vi "is_valid_ref.vi"(7 "raise error if invalid? (False)":bool, 8 "error in (no error)":errorcluster, 11 "Table in":refnum<class "Table.lvclass">) -> (0 "error out":errorcluster, 2 "is_valid_ref?":bool, 3 "Table out":refnum<class "Table.lvclass">)   [LabVIEW 2020, in "toml_edit.lvlib" / "Table.lvclass"]
uses:
  Table.lvclass
  Table.lvclass/Table.ctl
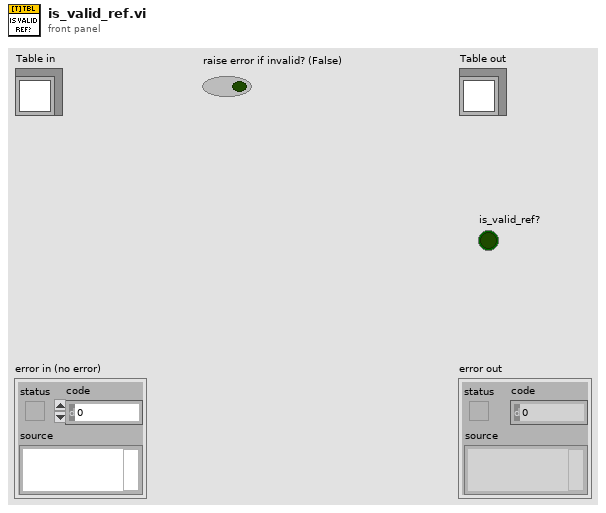
[diagram p1: front panel]
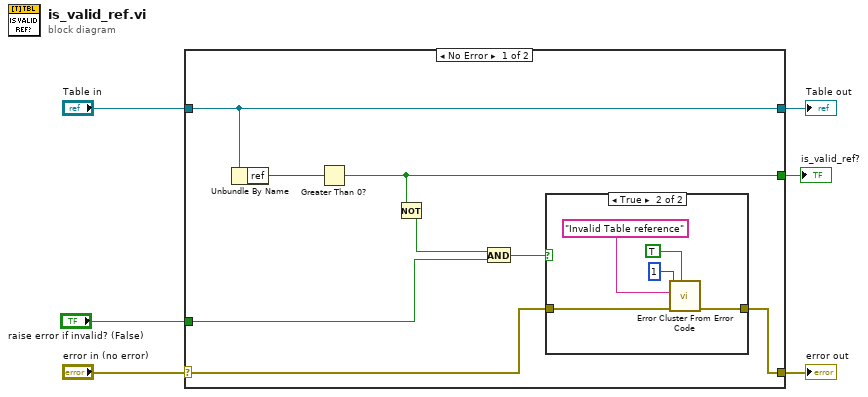
[diagram p0: block diagram]
diagram:
  n1 = case shown="No Error" "error in (no error)" {
    selector: "error in (no error)" -> [w8 w22]
    tunnel: [w7 w22] -> w5
    tunnel: [w14 w21] -> w3
    tunnel: "Table in" -> [w14 w21]
    tunnel: [w12 _] -> w2
    tunnel: "raise error if invalid? (False)" -> [w10 _]
    frame No Error {
      n2 = Unbundle By Name(w14) -> ("ref"=w13:u64)
      n3 = Greater Than 0?(x=w13) -> (x > 0?=w12:bool)
      n4 = Not(x=w12) -> (.not. x?=w11:bool)
      n5 = And(x=w11, y=w10) -> (x .and. y?=w9:bool)
      n6 = case shown="True" w9 {
        tunnel: [w15 w17] -> w7
        tunnel: w8 -> [w15 w16]
        frame False {
        }
        frame True {
          n7 = call <vilib>:"Error Cluster From Error Code.vi"("show call chain? (False)"=TRUE, "error in (no error)"=w16, "error message (\"\")"="Invalid Table reference" ("error message (\"\")"), "error code (0)"=1) -> ("error out"=w17:errorcluster)  [unwired: 5 in]
        }
      }
    }
    frame Error {
    }
  }
  "error out" <- w5
  "Table out" <- w3
  "is_valid_ref?" <- w2
